vi "RANGE Running Average.vi"(8 "Error In":errorcluster, 9 "Avg Interval (Sec)":i32, 10 "New Value":dbl, 11 "Array in":dbl[](array[numeric])) -> (0 "Error Out":errorcluster, 2 "Array out":dbl[](array[numeric]), 3 "Running Average":dbl)   [LabVIEW 2016]
uses:
  <vilib>/Analysis/baseanly.llb/Mean (DBL).vi
  <vilib>/Analysis/NI_AALBase.lvlib
panel:
  out "size(s)":i32
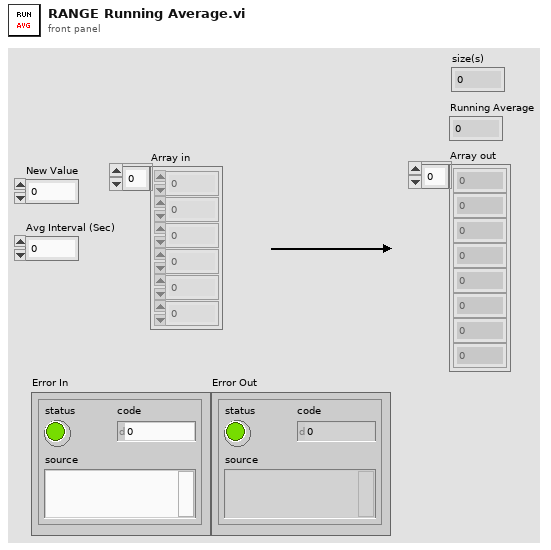
[diagram p1: front panel]
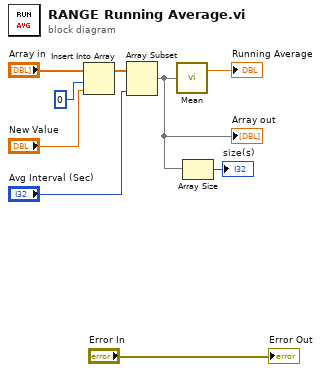
[diagram p0: block diagram]
diagram:
  n1 = Insert Into Array(array="Array in", index=0, new element="New Value") -> (w7:dbl[])
  n2 = Array Subset(array=w7, length="Avg Interval (Sec)") -> (w2:dbl[])  [unwired: 1 in]
  "Array out" <- w2
  n3 = call-poly <vilib>:"Mean.vi"("X"=w2) -> ("mean"=→"Running Average":dbl)  [unwired: 1 out]
  n4 = Array Size(array=w2) -> (size(s)=→"size(s)":i32)
  "Error Out" <- "Error In"
